vi "splitFractionalSeconds.vi"(10 "(Float) Time (s)":dbl format="%#.6f", 11 "Epoch in":refnum<class "Epoch.lvclass">) -> (1 "Fractional Second":dbl format="%#.6f", 2 "(Integer) Time (s)":i64, 3 "Epoch out":refnum<class "Epoch.lvclass">)   [LabVIEW 2013, in "Epoch.lvclass"]
uses:
  Epoch.lvclass
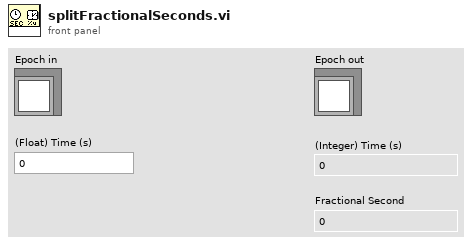
[diagram p1: front panel]
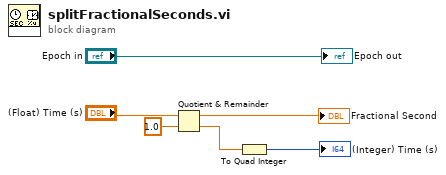
[diagram p0: block diagram]
diagram:
  n1 = Quotient & Remainder(x="(Float) Time (s)", y=1.0) -> (x-y*floor(x/y)=→"Fractional Second":dbl, floor(x/y)=w2:dbl)
  n2 = To Quad Integer(1:w2) -> (0:→"(Integer) Time (s)":i64)
  "Epoch out" <- "Epoch in"
